vi "fft_demod_update.vi"(4 "Current/sensor index":i32 min=0 max=1 step=1, 6 "Reset":bool, 10 "Config":T1={"IO params"={"Conversion"={"Rate"=4.0, "Num cards"=2, "Out channels"=4}, "Carriers"={"Phase shift"=180.0, "Levels"=[[0.8, 0.8, 0.8], [0.03, 0.03, 0.03]], "Delay samples"=73.15}, "TCP"={"Host"="192.168.1.15", "Port"=6666, "Buffering"=6, "Timeout"=6}, "Input channel sign"=[1, 1, 1]}, "High rate STFT"={"Win param"=101.5, "Window type"=61, "Win order"=2, "DFT size"=64, "Channels"=[7], "Oversample"=64}, "Low rate STFT"={"Win param"=120.0, "Window type"=61, "Win order"=8, "DFT size"=64, "Channels"=[7], "Oversample"=64}, "Filtering "=[]} {"Filtering"."Distortion"."Limit" format="%#_3p"; "Filtering"."Distortion"."LF cut" format="%#_3p"; "Filtering"."Kalman"."Measure noise" format="%#_3p"; "Filtering"."Kalman"."Process noise" format="%#_3p"; "Filtering"."Hum"."Limit" format="%#_3p"; "Filtering"."Hum"."Frequency" format="%#_4p"; "Low rate STFT"."Oversample" min=1 step=1; "Low rate STFT"."Channels" min=0 step=1; "Low rate STFT"."DFT size" min=1 step=1; "Low rate STFT"."Window type" items=["Rectangle"=0, "Hanning"=1, "Hamming"=2, "Blackman-Harris"=3, "Exact Blackman"=4, "Blackman"=5, "Flat Top"=6, "4 Term B-Harris "=7, "7 Term B-Harris"=8, "Low Sidelobe"=9, "Blackman Nuttall"=11, "Triangle"=30, "Bartlett-Hanning"=31, "Bohman"=32, "Parzen"=33, "Welch"=34, "Kaiser"=60, "Dolph-Chebyshev"=61, "Gaussian"=62]; "High rate STFT"."Oversample" min=1 step=1; "High rate STFT"."Channels" min=0 step=1; "High rate STFT"."DFT size" min=1 step=1; "High rate STFT"."Window type" items=["Rectangle"=0, "Hanning"=1, "Hamming"=2, "Blackman-Harris"=3, "Exact Blackman"=4, "Blackman"=5, "Flat Top"=6, "4 Term B-Harris "=7, "7 Term B-Harris"=8, "Low Sidelobe"=9, "Blackman Nuttall"=11, "Triangle"=30, "Bartlett-Hanning"=31, "Bohman"=32, "Parzen"=33, "Welch"=34, "Kaiser"=60, "Dolph-Chebyshev"=61, "Gaussian"=62]; "IO params"."Input channel sign" min=-1 max=1 step=1; "IO params"."Carriers"."Levels" min=0.0 step=0.1; "IO params"."Conversion"."Rate" format="%#_8g"}, 11 "Signal":dbl[](array[numeric])) -> (0 "Measure noise RMS":dbl[](array[numeric]) format="%#_2p", 2 "Measurement amplitudes":cdb[](array[numeric]) format="%_3p")   [LabVIEW 2026]
uses:
  ilemt_config.ctl
  system/IO_params.ctl
  stft_params.ctl
  <vilib>/Analysis/4window.llb/windowTd.ctl
  filter_params.ctl
  detrend_mode.ctl
  <vilib>/Analysis/NI_AALPro.lvlib
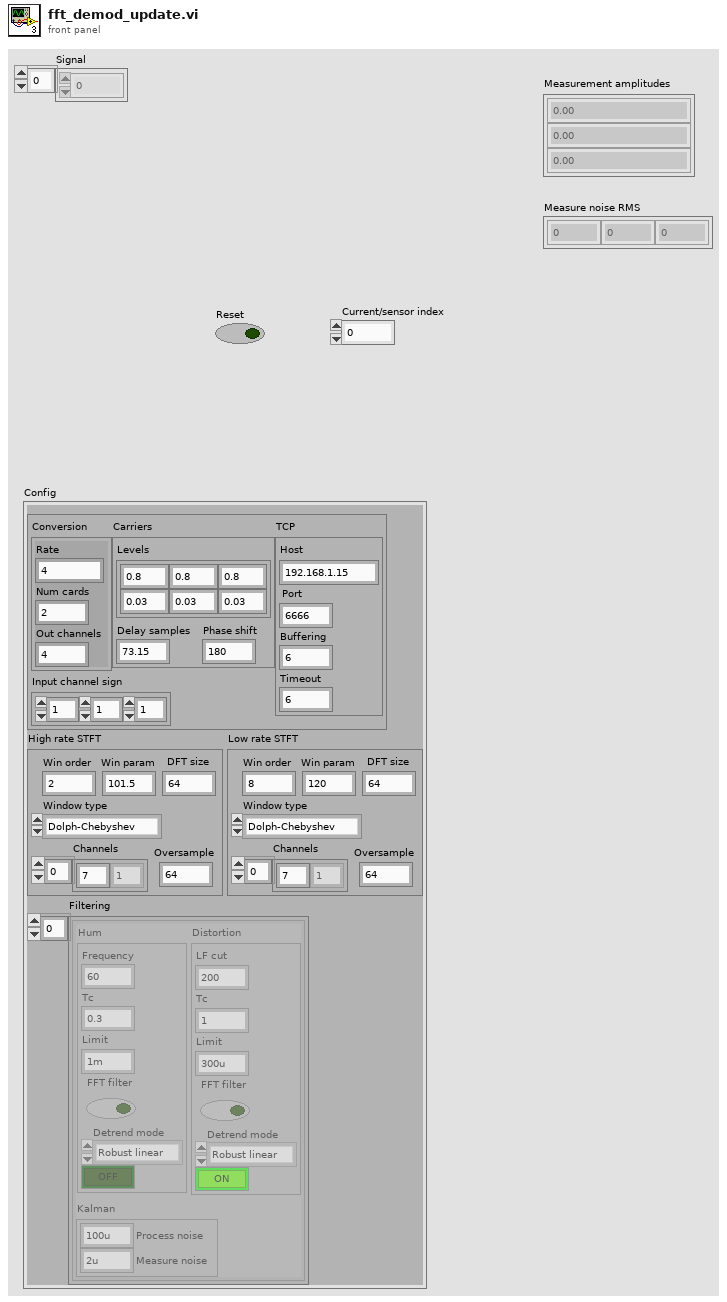
[diagram p1: front panel]
types:
  T1 = typedef "ilemt_config.ctl" = cluster{"IO params":T2, "High rate STFT":T3, "Low rate STFT":T3, "Filtering ":T5[]}
  T2 = typedef "IO_params.ctl" = cluster{"Conversion":cluster{"Rate":dbl, "Num cards":u32, "Out channels":u32}, "Carriers":cluster{"Phase shift":dbl, "Levels":dbl[][], "Delay samples":dbl}, "TCP":cluster{"Host":string, "Port":i32, "Buffering":u32, "Timeout":u32}, "Input channel sign":i32[]}
  T3 = typedef "stft_params.ctl" = cluster{"Win param":dbl, "Window type":T4, "Win order":i32, "DFT size":i32, "Channels":i32[], "Oversample":i32}
  T4 = typedef "NI_AALPro.lvlib/windowTd.ctl" = u32
  T5 = typedef "filter_params.ctl" = cluster{"Hum":cluster{"Frequency":dbl, "Tc":dbl, "Limit":dbl, "FFT filter":bool, "Detrend mode":T6, "Enable":bool}, "Kalman":cluster{"Process noise":dbl, "Measure noise":dbl}, "Distortion":cluster{"LF cut":dbl, "Tc":dbl, "Limit":dbl, "FFT filter":bool, "Detrend mode":T6, "Enable":bool}}
  T6 = typedef "detrend_mode.ctl" = enum16{"Zero mean", "Linear", "Robust linear"}
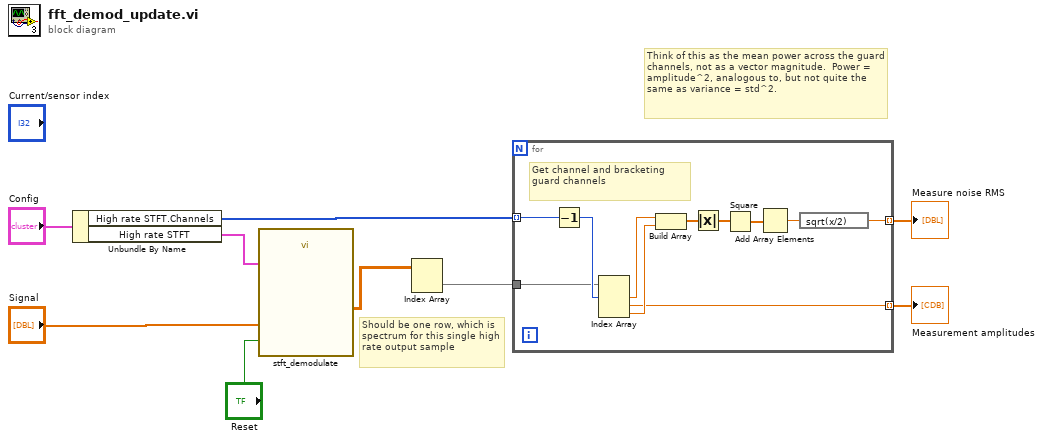
[diagram p0: block diagram]
diagram:
  # "Think of this as the mean power across the guard channels, not as a vector magnitude.  Power = amplitude^2, analogous to, but not quite the same as variance = std^2."
  # "Should be one row, which is spectrum for this single high rate output sample"
  n1 = Unbundle By Name("Config") -> ("High rate STFT.Channels"=w5:i32[], "High rate STFT"=w7:T3)
  n2 = call "stft_demodulate.vi"("STFT params"=w7, "Reset"="Reset", "X"="Signal") -> ("STFT"=w4:cdb[][])  [unwired: 6 in, 2 out]
  n3 = Index Array(array=w4) -> (element=w3:cdb[])  [unwired: 2 in]
  n4 = for {
    tunnel: [w13] -> w1 mode=indexing
    tunnel: w3 -> [w11]
    tunnel: w5 -> [w12] mode=indexing
    tunnel: [w10] -> w2 mode=indexing
    # "Get channel and bracketing guard channels"
    n5 = Decrement(x=w12) -> (x-1=w20:i32)
    n6 = Index Array(array=w11, index #1=w20) -> (element #1=w19:cdb, element #2=w13:cdb, element #3=w18:cdb)  [unwired: 2 in]
    n7 = Build Array(w19, w18) -> (w15:cdb[])
    n8 = Absolute Value(x=w15) -> (abs(x)=w14:dbl[])
    n9 = Square(x=w14) -> (x^2=w16:dbl[])
    n10 = Add Array Elements(numeric array=w16) -> (sum=w17:dbl)
    n11 = expression code="sqrt(x/2)"(w17) -> (w10:dbl)
  }
  "Measurement amplitudes" <- w1
  "Measure noise RMS" <- w2
